vi "Position to Voltage.vi"(10 "X Pos":dbl=192.0, 11 "X Parameters":T1={"Number of X Steps"=200, "Max X (V)"=2.0, "Min X (V)"=-2.0}) -> (3 "Voltage":dbl)   [LabVIEW 2011]
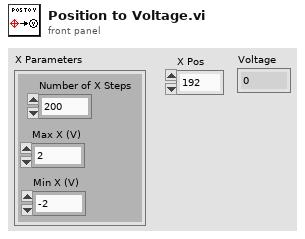
[diagram p1: front panel]
types:
  T1 = cluster{"Number of X Steps":i32, "Max X (V)":dbl, "Min X (V)":dbl}
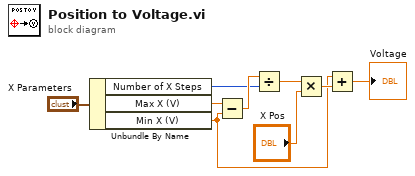
[diagram p0: block diagram]
diagram:
  n1 = Unbundle By Name("X Parameters") -> ("Number of X Steps"=w5:i32, "Max X (V)"=w4:dbl, "Min X (V)"=w2:dbl)
  n2 = Subtract(x=w4, y=w2) -> (x-y=w9:dbl)
  n3 = Divide(x=w9, y=w5) -> (x/y=w7:dbl)
  n4 = Multiply(x=w7, y="X Pos") -> (x*y=w6:dbl)
  n5 = Add(x=w2, y=w6) -> (x+y=→"Voltage":dbl)
